vi "voltage_to_distance(SubVI).vi"(11 "Voltage(V)":dbl) -> (3 "distance (cm)":dbl)   [LabVIEW 2019]
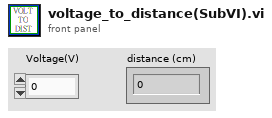
[diagram p1: front panel]
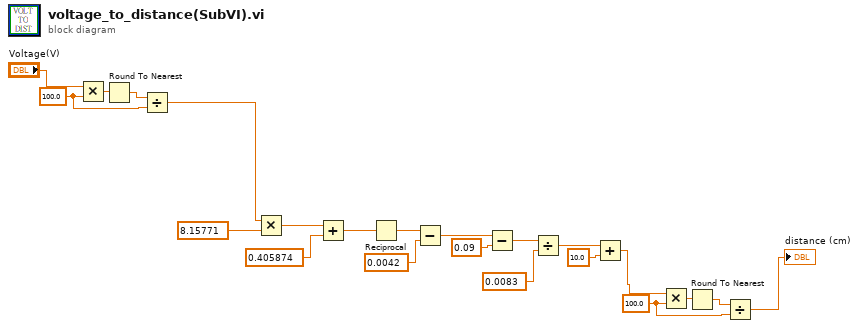
[diagram p0: block diagram]
diagram:
  w5 = 100.0 ("y")
  w7 = 100.0 ("y")
  n1 = Multiply(x="Voltage(V)", y=w7) -> (x*y=w9:dbl)
  n2 = Round To Nearest(number=w9) -> (nearest integer value=w8:dbl)
  n3 = Divide(x=w8, y=w7) -> (x/y=w6:dbl)
  n4 = Multiply(x=w6, y=8.15771 ("m")) -> (x*y=w22:dbl)
  n5 = Add(x=w22, y=0.405874 ("k")) -> (x+y=w21:dbl)
  n6 = Reciprocal(x=w21) -> (1/x=w20:dbl)
  n7 = Subtract(x=w20, y=0.0042 ("s")) -> (x-y=w17:dbl)
  n8 = Subtract(x=w17, y=0.09) -> (x-y=w19:dbl)
  n9 = Divide(x=w19, y=0.0083) -> (x/y=w18:dbl)
  n10 = Add(x=w18, y=10.0) -> (x+y=w2:dbl)
  n11 = Multiply(x=w2, y=w5) -> (x*y=w3:dbl)
  n12 = Round To Nearest(number=w3) -> (nearest integer value=w4:dbl)
  n13 = Divide(x=w4, y=w5) -> (x/y=→"distance (cm)":dbl)
